vi "FPGAcode_check_values.vi"() -> ()   [LabVIEW 2015]
uses:
  <vilib>/Platform/TimedLoop/XDataNode/wakeup.ctl
  <vilib>/Platform/TimedLoop/XDataNode/XDNodeRunTimeDep.lvlib
  <vilib>/Platform/TimedLoop/XDataNode/nitl_modes.ctl
  <vilib>/Platform/TimedLoop/XDataNode/timing_clust.ctl
  <vilib>/Platform/TimedLoop/XDataNode/XDataNode.xnode
  <vilib>/eio/EIONode/EIONode.xnode
  <vilib>/rvi/eio/common/nirviEmuTemplateMethod_errors.vi
panel:
  out "Check Data?":bool
  out "Filter":i16
  out "Wait time 7":i32
  out "Wait time 6":i32
  out "delay 7":i32
  out "delay 6":i32
  out "Vel Count 7":i32
  out "Vel Count 6":i32
  out "Wait time 5":i32
  out "delay 5":i32
  out "Vel Count 5":i32
  out "Vel Count 4":i32
  out "delay 4":i32
  out "Wait time 4":i32
  out "Vel Count 3":i32
  out "delay 3":i32
  out "Wait time 3":i32
  out "Wait time 2":i32
  out "delay 2":i32
  out "Vel Count 2":i32
  out "Wait time 1":i32
  out "delay 1":i32
  out "Vel Count 1":i32
  out "Filter 1 Detector 3 Correlation":i32
  in  "Filter 2 threshold":i32=1000
  out "Filter 2 Detector 3 Correlation":i32
  in  "Filter 1 threshold":i32=1000
  in  "Filter 3 threshold":i32=1000
  out "Filter 3 Detector 3 Correlation":i32
  in  "Filter 4 threshold":i32=1000
  out "Filter 4 Detector 3 Correlation":i32
  in  "Filter 5 threshold":i32
  out "Filter 5 Detector 3 Correlation":i32
  in  "Filter 6 threshold":i32
  out "Filter 6 Detector 3 Correlation":i32
  in  "Filter 7 threshold":i32
  out "Filter 7 Detector 3 Correlation":i32
  out "Plates":bool
  in  "High Charge Limit":i16
  in  "Low Charge Limit":i16
  in  "High Velocity Count":i32
  in  "Low Velocity Count":i32
  in  "High Mass Limit":i64
  in  "Low Mass Limit":i64
  in  "Mult1":fxp<+,16,7>
  out "Delay1":bool
  in  "One Shot":bool
  out "Not Armed?":bool
  in  "Reset One Shot":bool
  out "Del Not Armed?":bool
  out "IO Module\\AI 0":i16
  out "IO Module\\AI 1":i16
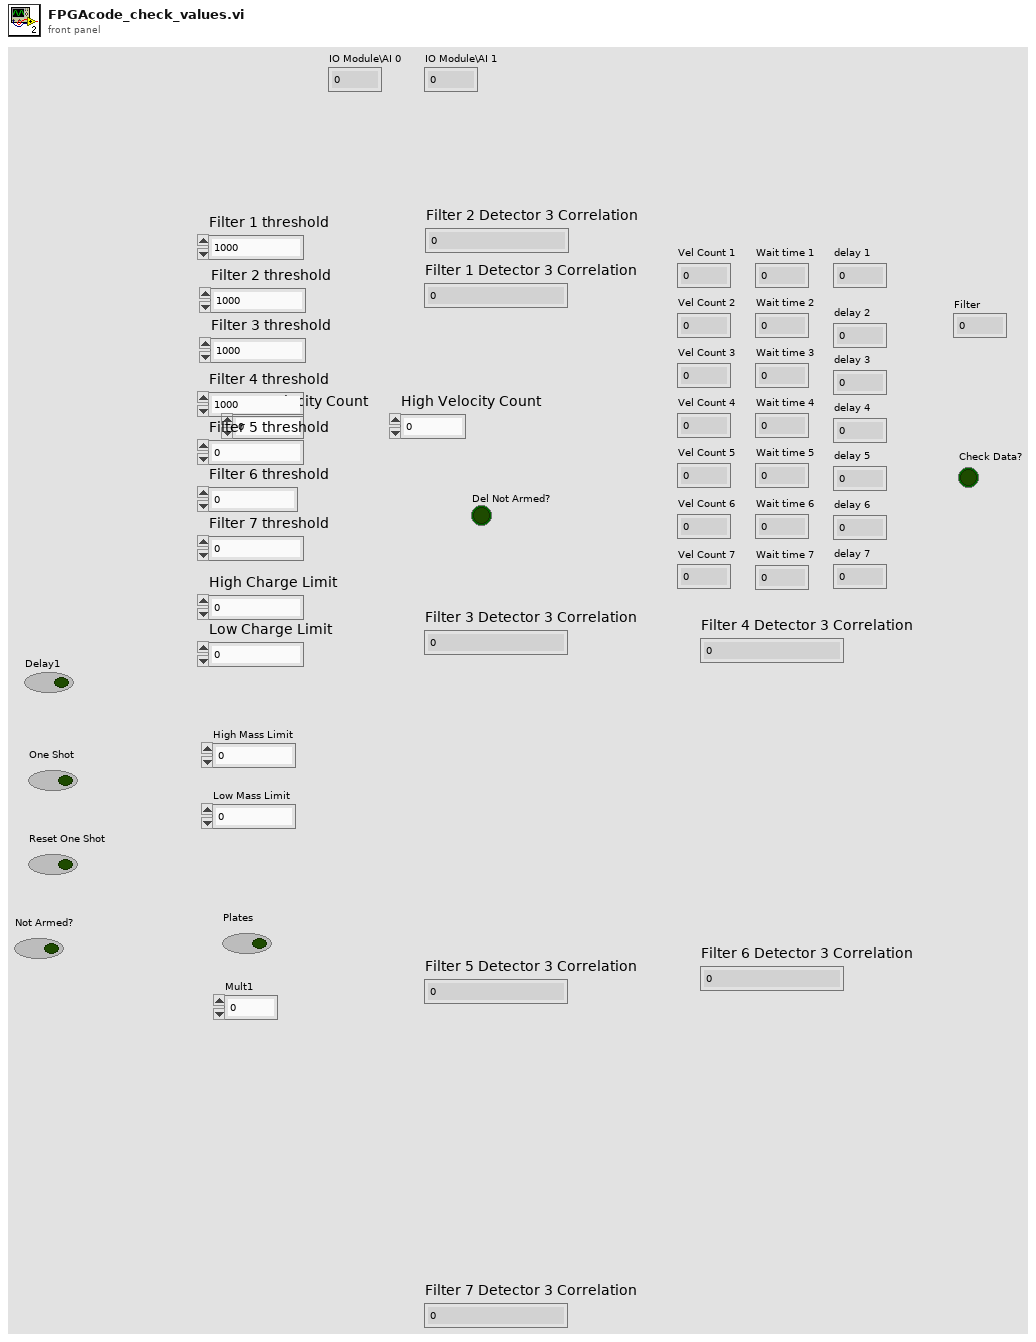
[diagram p1: front panel]
types:
  T1 = typedef "XDNodeRunTimeDep.lvlib/timing_clust.ctl" = cluster{"Expected End [f-1]":u64, "Actual End [f-1]":u64, "Finished Late? [f-1]":bool, "Expected End [i-1]":u64, "Actual End [i-1]":u64, "Finished Late? [i-1]":bool, "Expected Start [i]":u64, "Actual Start [i]":u64, "Expected Start [f]":u64, "Actual Start [f]":u64, "Source Name":string, "Structure Name":string, "Period":i64, "Deadline":i64, "Offset":i64, "Start":i64, "Priority":i32, "Timeout":i32, "Mode":T2, "Wakeup Reason":T3, "Error":errorcluster, "Source Type":string, "Secondary Source Type":string, "Global End Time":u64, "Global Start Time":u64, "Frame Duration":u64, "Iteration Duration":u64, "Assigned CPU":i32, "I/O Scan Engine Mode":u32}
  T2 = typedef "XDNodeRunTimeDep.lvlib/nitl_modes.ctl" = enum32{"No Change", "Process missed periods, maintain original phase", "Discard missed periods, maintain original phase", "Process missed periods, ignore original phase", "Discard missed periods, ignore original phase"}
  T3 = typedef "XDNodeRunTimeDep.lvlib/wakeup.ctl" = enum32{"Normal", "Aborted", "Asynchronous wakeup", "Timing source error", "Timed loop error", "Timeout"}
  T4 = cluster{"Separation cut off 1":i32, "Filter Number":i32, "Separation cut off 2":i32}
  T5 = cluster{"Old Average":i32, "New Average":i32, "Current State":u8, "Detector 1 Correlation":i32, "Detector 3 Correlation":i32, "Velocity Count":i32, "Detector Counter in":i32, "Timeout Count in":i32, "Measured Charge in":i32, "Filter Threshold":i32, "High Correlation in":i32, "Offset":i32, "Offset Average":i32, "Measured Velocity In":i32, "Mult Cluster":cluster{"Mult1":fxp<+,16,7>, "Mult1 Use?":bool}, "Final Delay Count In":u16, "Delay1 In":i32}
  T6 = cluster{"High Charge Limit":i16, "Low Charge Limit":i16, "Low Velocity Count":i32, "High Velocity Count":i32, "Low Velocity Count":i32, fxp<+,30,25>, "High Mass Limit":i64, "Low Mass Limit":i64}
  T7 = cluster{"Average Out":i32, "Next State":u8, "Velocity Count out":i32, "Detector counter out":i32, "Timeout count out":u32, "Measured Charge Out":i32, "High Correlation Out":i32, "Plates":bool, "Offset Out":i32, "Measured Velocity Out":i32, "Final Delay Count Out":u16, "Out1":bool, "Delay1":i32}
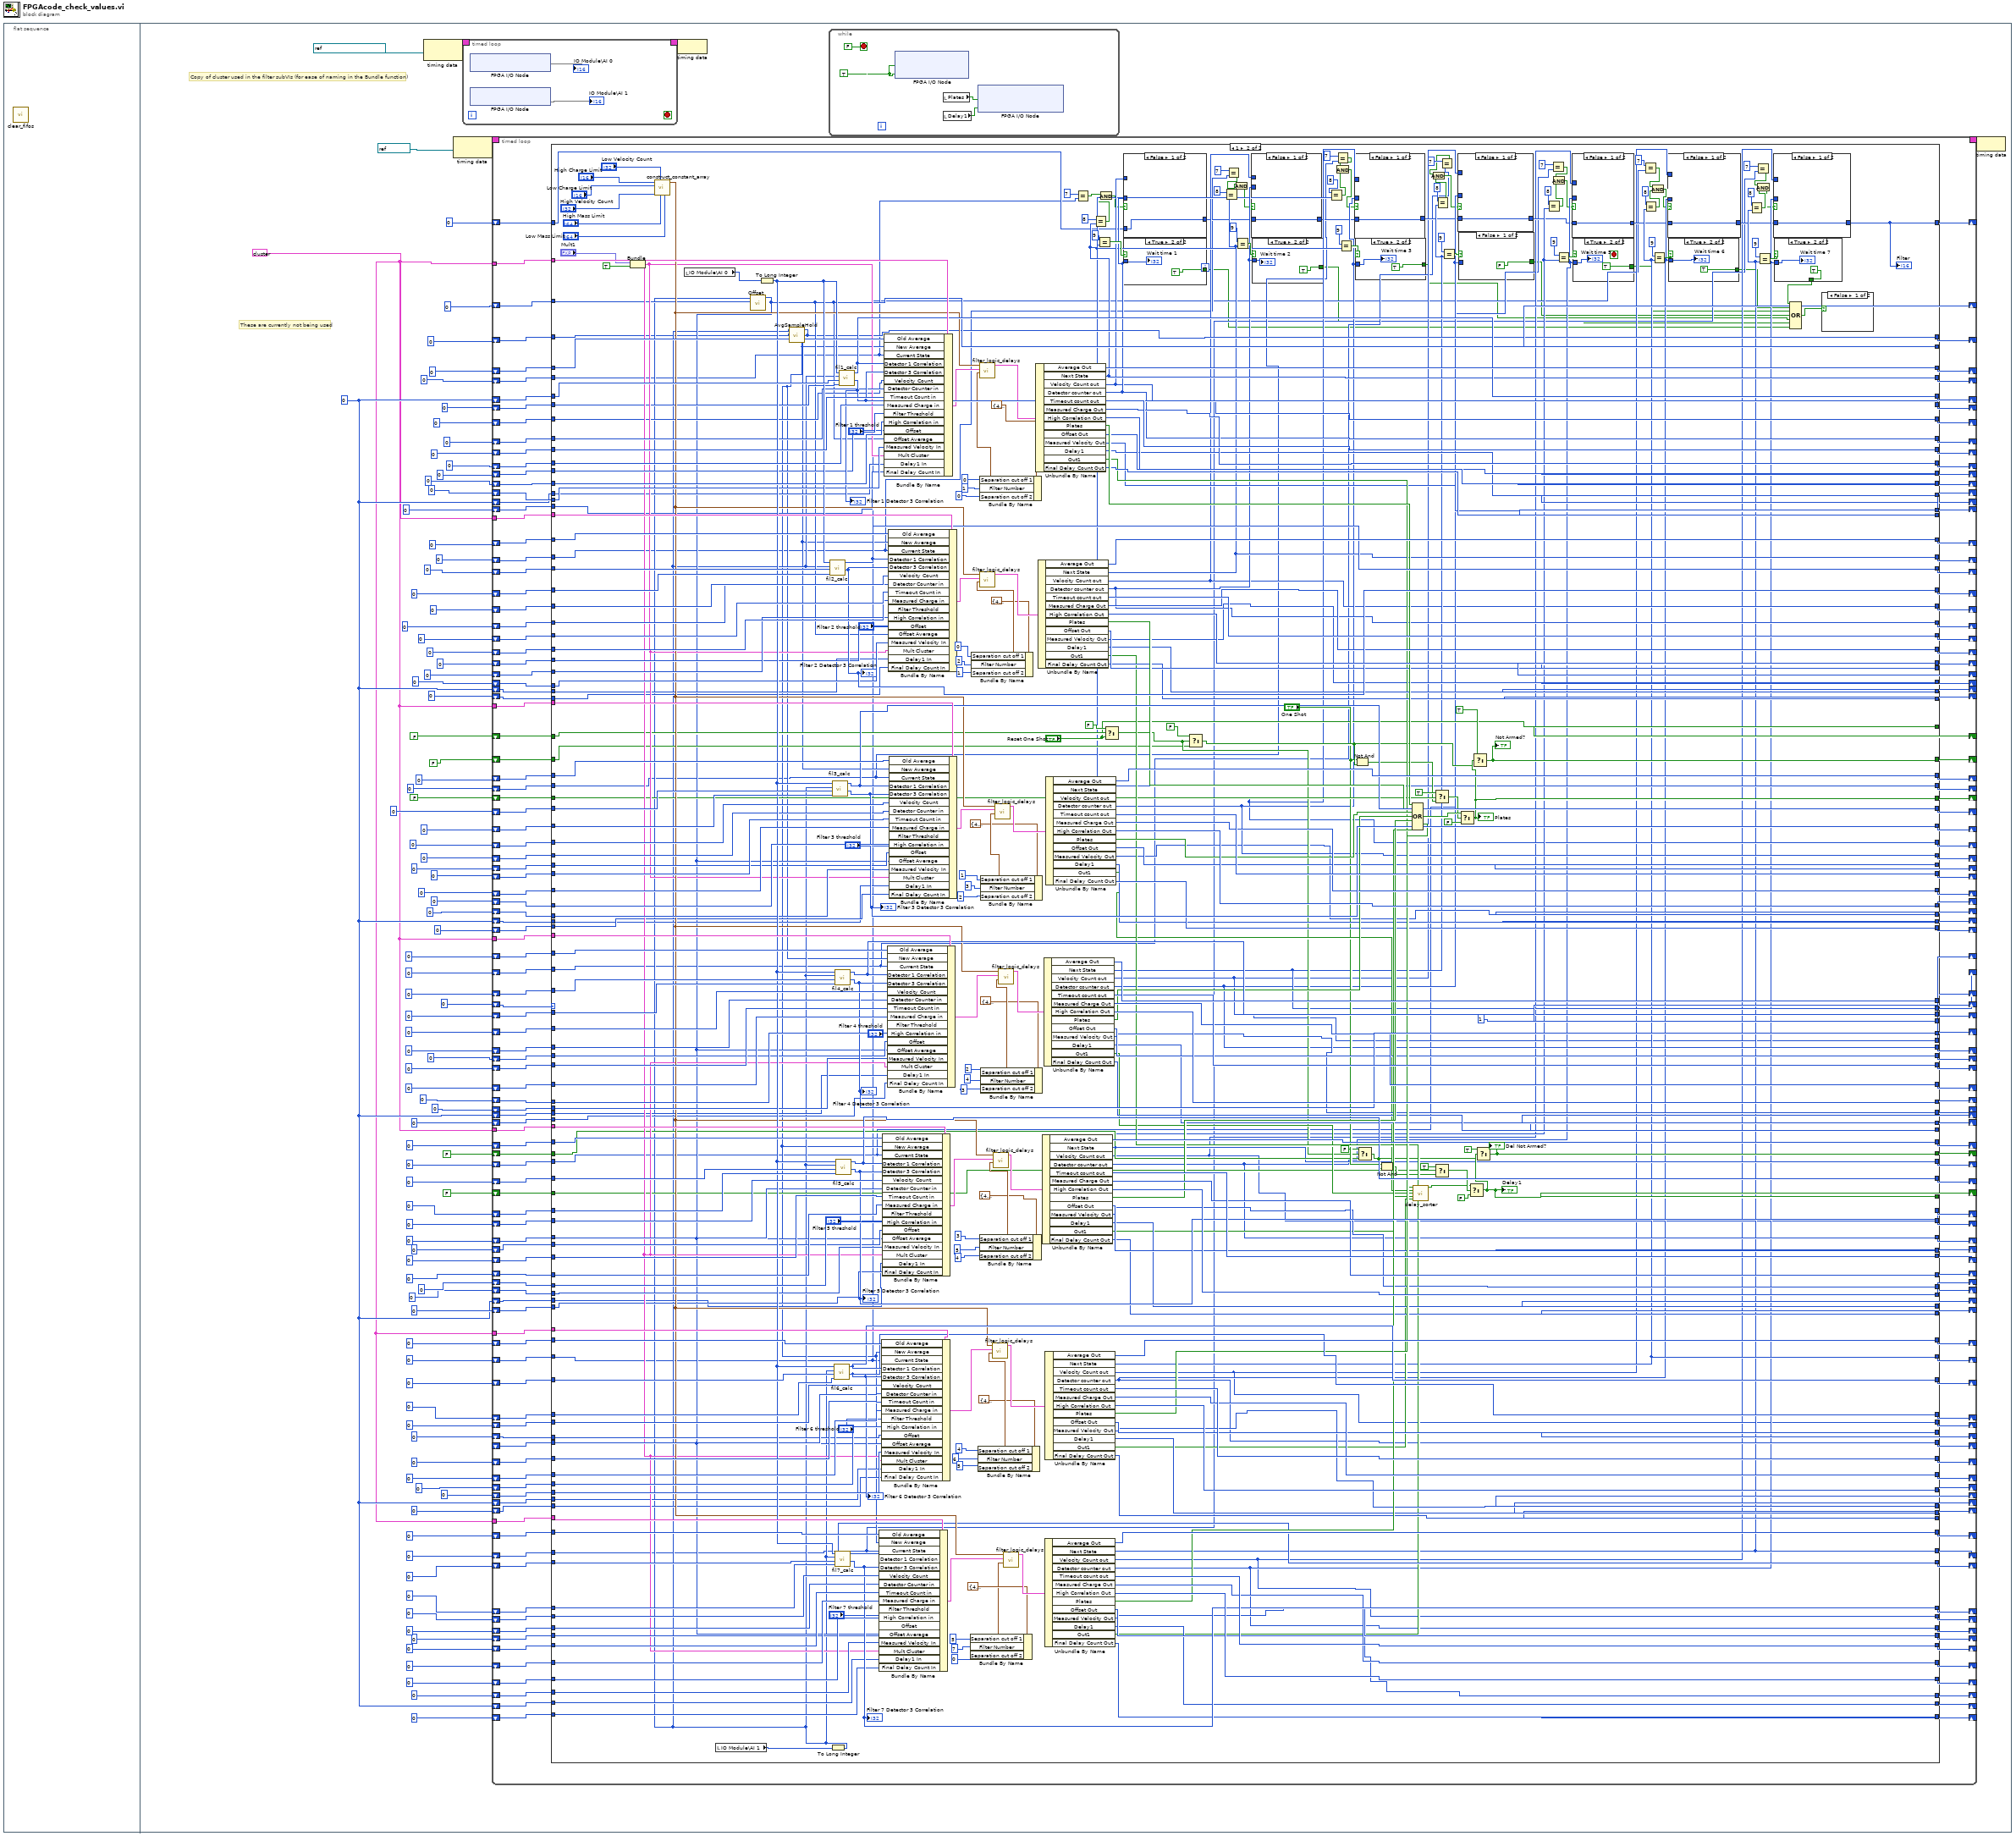
[diagram p0: block diagram]
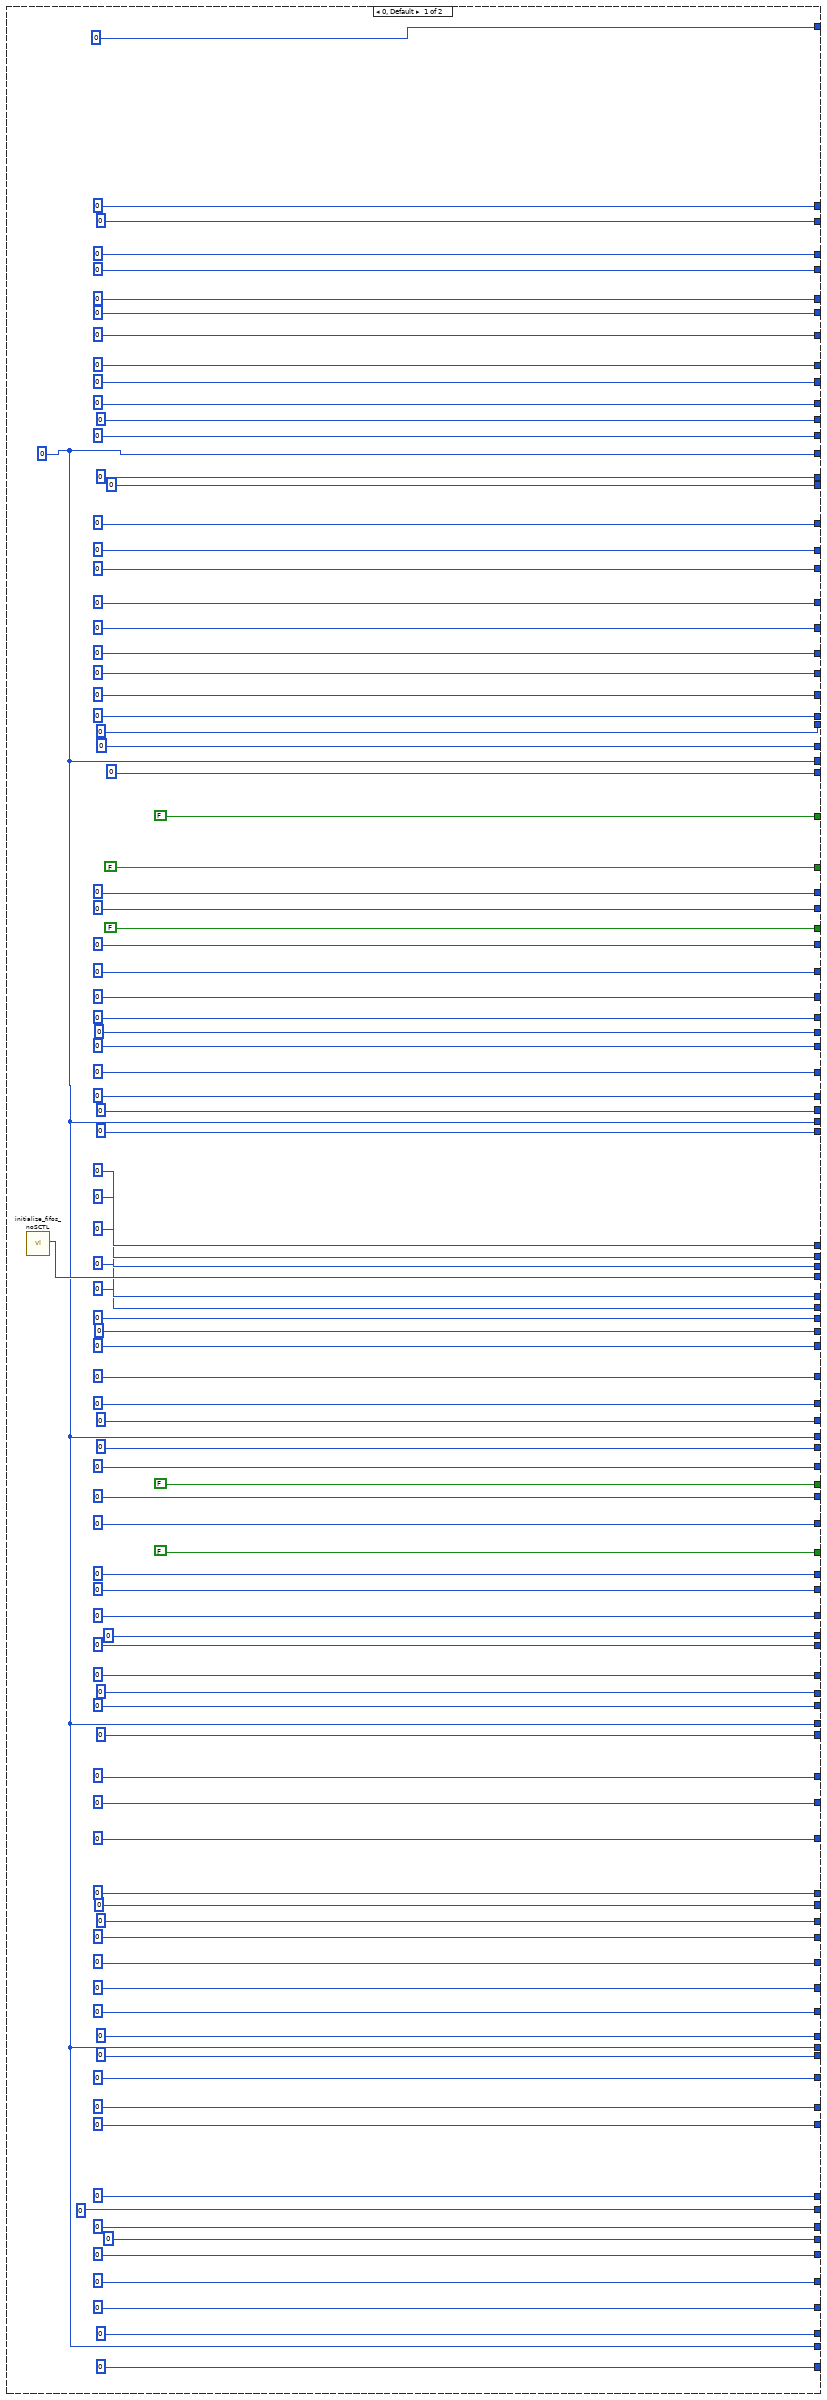
[diagram p2: hidden frame]
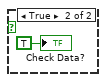
[diagram p3: hidden frame]
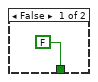
[diagram p4: hidden frame]
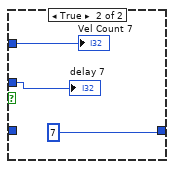
[diagram p5: hidden frame]
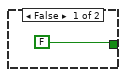
[diagram p6: hidden frame]
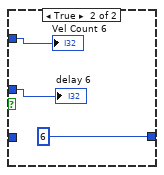
[diagram p7: hidden frame]
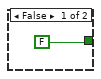
[diagram p8: hidden frame]
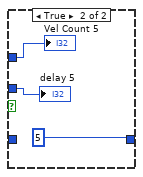
[diagram p9: hidden frame]
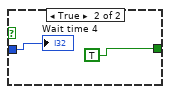
[diagram p10: hidden frame]
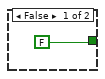
[diagram p11: hidden frame]
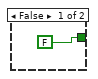
[diagram p12: hidden frame]
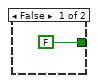
[diagram p13: hidden frame]
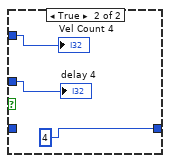
[diagram p14: hidden frame]
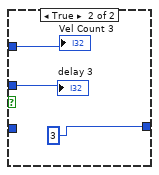
[diagram p15: hidden frame]
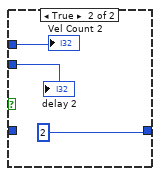
[diagram p16: hidden frame]
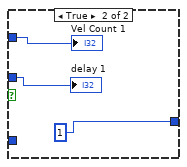
[diagram p17: hidden frame]
diagram:
  n1 = flat-sequence {
    frame #0 {
      n2 = call "clear_fifos.vi"() -> ()  [unwired: 1 in]
    }
    frame #1 {
      w6 = T5 {"Old Average"=0, "New Average"=0, "Current State"=0, "Detector 1 Correlation"=0, "Detector 3 Correlation"=0, "Velocity Count"=0, "Detector Counter in"=0, "Timeout Count in"=0, "Measured Charge in"=0, "Filter Threshold"=0, "High Correlation in"=0, "Offset"=0, "Offset Average"=0, "Measured Velocity In"=0, "Mult Cluster"={"Mult1"=0.0, "Mult1 Use?"=FALSE}, "Final Delay Count In"=0, "Delay1 In"=0} ("Variables Cluster")
      w9 = 0 ("Detector 1 Correlation Out")
      # "These are currently not being used"
      # "Copy of cluster used in the filter subVIs (for ease of naming in the Bundle function)"
      n3 = node-c288(refnum<k21> "IO Module\\Data Clock" ("Source Name")) -> (w35:T1)
      n4 = node-c288(refnum<k21> "26MHz" ("Source Name")) -> (w99:T1)
      n5 = timed-loop {
        timing: w35 -> [_]
        timing-out: [_] -> w34
        stop <- _ stop-if-true
        n6 = xnode "FPGA I/O Node"() -> ("IO Module\\AI 0 Data N"=→"IO Module\\AI 0")  [unwired: 1 in, 1 out]
        n7 = xnode "FPGA I/O Node"() -> ("IO Module\\AI 1 Data N"=→"IO Module\\AI 1")  [unwired: 1 in, 1 out]
      }
      n8 = timed-loop {
        timing: w99 -> [_]
        timing-out: [_] -> w98
        shift-right: [w311] -> _
        shift-left: 0 ("Velocity Count out") -> [w233]
        shift-right: [w312] -> _
        shift-left: 0 ("Detector 1 Correlation out") -> [w234]
        shift-right: [w198] -> _
        shift-left: 0 ("Detector counter out") -> [w235]
        shift-right: [w229] -> _
        shift-left: 0 ("Next State") -> [w236]
        shift-right: [w197] -> _
        shift-left: 0 ("Detector 3 Correlation out") -> [w232]
        shift-right: [w310] -> _
        shift-left: 0 ("Timeout count out") -> [w231]
        shift-right: [w225] -> _
        shift-left: 0 ("Next State") -> [w228]
        shift-right: [w224] -> _
        shift-left: 0 ("Detector counter out") -> [w227]
        shift-right: [w196] -> _
        shift-left: 0 ("Detector 1 Correlation out") -> [w304]
        shift-right: [w301] -> _
        shift-left: 0 ("Velocity Count out") -> [w303]
        shift-right: [w300] -> _
        shift-left: u32 0 ("Detector 3 Correlation out") -> [w302]
        shift-right: [w295] -> _
        shift-left: 0 ("Timeout count out") -> [w296]
        shift-right: [w219] -> _
        shift-left: 0 ("Next State") -> [w222]
        shift-right: [w194] -> _
        shift-left: 0 ("Detector counter out") -> [w292]
        shift-right: [w290] -> _
        shift-left: 0 ("Detector 1 Correlation out") -> [w291]
        shift-right: [w288] -> _
        shift-left: u32 0 ("Velocity Count out") -> [w289]
        shift-right: [w193] -> _
        shift-left: 0 ("Detector 3 Correlation out") -> [w287]
        shift-right: [w286] -> _
        shift-left: 0 ("Timeout count out") -> [w221]
        shift-right: [w313] -> _
        shift-left: u8 0 ("High Correlation Out") -> [w316]
        shift-right: [w305] -> _
        shift-left: u8 0 ("High Correlation Out") -> [w306]
        shift-right: [w220] -> _
        shift-left: 0 ("High Correlation Out") -> [w223]
        shift-right: [w314] -> _
        shift-left: 0 ("Measured Charge Out") -> [w317]
        shift-right: [w307] -> _
        shift-left: 0 ("Measured Charge Out") -> [w308]
        shift-right: [w294] -> _
        shift-left: u8 0 ("Measured Charge Out") -> [w293]
        shift-right: [w184] -> _
        shift-left: 0 ("Output New Average") -> [w318]
        shift-right: [w230] -> _
        shift-left: w9 -> [w237]
        tunnel: w6 -> [w315]
        shift-right: [w195] -> _
        shift-left: 0 ("High Sample Out") -> [w298]
        shift-right: [w299] -> _
        shift-left: 0 ("High Correlation Out") -> [w226]
        tunnel: w6 -> [w309]
        tunnel: w6 -> [w297]
        shift-right: [w285] -> _
        shift-left: 0 ("Average Out") -> [w284]
        shift-right: [w283] -> _
        shift-left: u8 0 ("Next State") -> [w282]
        shift-right: [w215] -> _
        shift-left: 0 ("Detector 1 Correlation out") -> [w217]
        shift-right: [w214] -> _
        shift-left: 0 ("Detector 3 Correlation out") -> [w216]
        shift-right: [w192] -> _
        shift-left: 0 ("Velocity Count out") -> [w281]
        shift-right: [w280] -> _
        shift-left: 0 ("Detector counter out") -> [w279]
        shift-right: [w278] -> _
        shift-left: u32 0 ("Timeout count out") -> [w277]
        shift-right: [w191] -> _
        shift-left: 0 ("Measured Charge Out") -> [w276]
        shift-right: [w275] -> _
        shift-left: 0 ("High Correlation Out") -> [w218]
        tunnel: w6 -> [w274]
        shift-right: [w272] -> _
        shift-left: 0 ("Average Out") -> [w271]
        shift-right: [w270] -> _
        shift-left: u8 0 ("Next State") -> [w269]
        shift-right: [w210] -> _
        shift-left: 0 ("Detector 1 Correlation out") -> [w213]
        shift-right: [w209] -> _
        shift-left: 0 ("Detector 3 Correlation out") -> [w212]
        shift-right: [w190] -> _
        shift-left: 0 ("Velocity Count out") -> [w268]
        shift-right: [w267] -> _
        shift-left: 0 ("Detector counter out") -> [w266]
        shift-right: [w265] -> _
        shift-left: u32 0 ("Timeout count out") -> [w264]
        shift-right: [w189] -> _
        shift-left: 0 ("Measured Charge Out") -> [w263]
        shift-right: [w262] -> _
        shift-left: 0 ("High Correlation Out") -> [w211]
        tunnel: w6 -> [w273]
        shift-right: [w260] -> _
        shift-left: 0 ("Average Out") -> [w258]
        shift-right: [w259] -> _
        shift-left: u8 0 ("Next State") -> [w255]
        shift-right: [w205] -> _
        shift-left: 0 ("Detector 1 Correlation out") -> [w208]
        shift-right: [w204] -> _
        shift-left: 0 ("Detector 3 Correlation out") -> [w207]
        shift-right: [w187] -> _
        shift-left: 0 ("Velocity Count out") -> [w257]
        shift-right: [w254] -> _
        shift-left: _ -> [w256]
        shift-right: [w253] -> _
        shift-left: u32 0 ("Timeout count out") -> [w252]
        shift-right: [w188] -> _
        shift-left: 0 ("Measured Charge Out") -> [w251]
        shift-right: [w250] -> _
        shift-left: 0 ("High Correlation Out") -> [w206]
        tunnel: w6 -> [w261]
        shift-right: [w248] -> _
        shift-left: 0 ("Average Out") -> [w247]
        shift-right: [w246] -> _
        shift-left: u8 0 ("Next State") -> [w238]
        shift-right: [w200] -> _
        shift-left: 0 ("Detector 1 Correlation out") -> [w203]
        shift-right: [w199] -> _
        shift-left: 0 ("Detector 3 Correlation out") -> [w202]
        shift-right: [w186] -> _
        shift-left: 0 ("Velocity Count out") -> [w245]
        shift-right: [w244] -> _
        shift-left: 0 ("Detector counter out") -> [w243]
        shift-right: [w242] -> _
        shift-left: u32 0 ("Timeout count out") -> [w241]
        shift-right: [w185] -> _
        shift-left: 0 ("Measured Charge Out") -> [w240]
        shift-right: [w239] -> _
        shift-left: 0 ("High Correlation Out") -> [w201]
        tunnel: w6 -> [w249]
        shift-right: [w182] -> _
        shift-left: i16 0 -> [w183]
        shift-right: [w180] -> _
        shift-left: 0 -> [w181]
        shift-right: [w179] -> _
        shift-left: 0 -> [w176]
        shift-right: [w177] -> _
        shift-left: 0 -> [w178]
        shift-right: [w174] -> _
        shift-left: 0 ("Offset Out") -> [w175]
        shift-right: [w173] -> _
        shift-left: 0 ("Offset Out") -> [w172]
        shift-right: [w171] -> _
        shift-left: 0 ("Offset Out") -> [w170]
        shift-right: [w169] -> _
        shift-left: 0 ("Offset Out") -> [w168]
        shift-right: [w167] -> _
        shift-left: 0 ("Offset Out") -> [w166]
        shift-right: [w164] -> _
        shift-left: 0 -> [w165]
        shift-right: [w163] -> _
        shift-left: 0 -> [w152]
        shift-right: [w162] -> _
        shift-left: 0 -> [w153]
        shift-right: [w161] -> _
        shift-left: 0 -> [w154]
        shift-right: [w160] -> _
        shift-left: 0 -> [w155]
        shift-right: [w159] -> _
        shift-left: 0 -> [w156]
        shift-right: [w158] -> _
        shift-left: 0 ("Measured Velocity Out") -> [w157]
        shift-right: [w151] -> _
        shift-left: w9 -> [w149]
        shift-right: [w150] -> _
        shift-left: u32 0 ("Final Delay Count Out") -> [w148]
        shift-right: [w147] -> _
        shift-left: w9 -> [w145]
        shift-right: [w146] -> _
        shift-left: u32 0 ("Final Delay Count Out") -> [w144]
        shift-right: [w143] -> _
        shift-left: w9 -> [w141]
        shift-right: [w142] -> _
        shift-left: u32 0 ("Final Delay Count Out") -> [w140]
        shift-right: [w139] -> _
        shift-left: w9 -> [w137]
        shift-right: [w138] -> _
        shift-left: u32 0 ("Final Delay Count Out") -> [w136]
        shift-right: [w135] -> _
        shift-left: w9 -> [w133]
        shift-right: [w134] -> _
        shift-left: u32 0 ("Final Delay Count Out") -> [w132]
        shift-right: [w131] -> _
        shift-left: w9 -> [w129]
        shift-right: [w130] -> _
        shift-left: u32 0 ("Final Delay Count Out") -> [w128]
        shift-right: [w127] -> _
        shift-left: w9 -> [w125]
        shift-right: [w126] -> _
        shift-left: u32 0 ("Final Delay Count Out") -> [w124]
        shift-right: [w122] -> _
        shift-left: FALSE -> [w123]
        shift-right: [w121] -> _
        shift-left: FALSE ("f") -> [w120]
        shift-right: [w119] -> _
        shift-left: FALSE ("Reset One Shot") -> [w118]
        shift-right: [w114] -> _
        shift-left: FALSE -> [w117]
        shift-right: [w115] -> _
        shift-left: FALSE -> [w116]
        shift-right: [w113] -> _
        shift-left: i16 0 ("Filter") -> [w112]
        stop <- _ stop-if-true
        n9 = case shown="1" w183 {
          tunnel: w318 -> [_ w510]
          tunnel: w317 -> [_ w784]
          tunnel: w316 -> [_ w427]
          tunnel: w315 -> [_ w783]
          tunnel: [0 ("Average Out") w782] -> w314
          tunnel: [u16 0 ("Next State") w506] -> w313
          tunnel: [0 ("Detector counter out") w498] -> w312
          tunnel: [u32 0 ("Timeout count out") w781] -> w311
          tunnel: [0 ("High Correlation Out") w780] -> w310
          tunnel: w309 -> [_ w779]
          tunnel: w308 -> [_ w778]
          tunnel: [0 ("Average Out") w777] -> w307
          tunnel: w306 -> [_ w426]
          tunnel: [u16 0 ("Next State") w496] -> w305
          tunnel: w304 -> [_ w776]
          tunnel: w303 -> [_ w638]
          tunnel: w302 -> [_ w775]
          tunnel: [0 ("Detector counter out") w495] -> w301
          tunnel: [u32 0 ("Timeout count out") w774] -> w300
          tunnel: [0 ("High Correlation Out") w773] -> w299
          tunnel: w298 -> [_ w772]
          tunnel: w297 -> [_ w771]
          tunnel: w296 -> [_ w770]
          tunnel: [0 ("Average Out") w769] -> w295
          tunnel: [u16 0 ("Next State") w493] -> w294
          tunnel: w293 -> [_ w425]
          tunnel: w292 -> [_ w768]
          tunnel: w291 -> [_ w637]
          tunnel: [0 ("Detector counter out") w492] -> w290
          tunnel: w289 -> [_ w767]
          tunnel: [u32 0 ("Timeout count out") w766] -> w288
          tunnel: w287 -> [_ w765]
          tunnel: [0 ("High Correlation Out") w764] -> w286
          tunnel: [0 ("Average Out") w763] -> w285
          tunnel: w284 -> [_ w762]
          tunnel: [u16 0 ("Next State") w478] -> w283
          tunnel: w282 -> [_ w424]
          tunnel: w281 -> [_ w761]
          tunnel: [0 ("Detector counter out") w477] -> w280
          tunnel: w279 -> [_ w636]
          tunnel: [u32 0 ("Timeout count out") w760] -> w278
          tunnel: w277 -> [_ w759]
          tunnel: w276 -> [_ w758]
          tunnel: [0 ("High Correlation Out") w757] -> w275
          tunnel: w274 -> [_ w756]
          tunnel: w273 -> [_ w755]
          tunnel: [0 ("Average Out") w754] -> w272
          tunnel: w271 -> [_ w753]
          tunnel: [u16 0 ("Next State") w476] -> w270
          tunnel: w269 -> [_ w423]
          tunnel: w268 -> [_ w752]
          tunnel: [0 ("Detector counter out") w473] -> w267
          tunnel: w266 -> [_ w635]
          tunnel: [u32 0 ("Timeout count out") w751] -> w265
          tunnel: w264 -> [_ w750]
          tunnel: w263 -> [_ w749]
          tunnel: [0 ("High Correlation Out") w748] -> w262
          tunnel: w261 -> [_ w747]
          tunnel: [0 ("Average Out") w746] -> w260
          tunnel: [u16 0 ("Next State") w472] -> w259
          tunnel: w258 -> [_ w745]
          tunnel: w257 -> [_ w744]
          tunnel: w256 -> [_ w634]
          tunnel: w255 -> [_ w422]
          tunnel: [0 ("Detector counter out") w471] -> w254
          tunnel: [u32 0 ("Timeout count out") w743] -> w253
          tunnel: w252 -> [_ w742]
          tunnel: w251 -> [_ w741]
          tunnel: [0 ("High Correlation Out") w740] -> w250
          tunnel: w249 -> [_ w739]
          tunnel: [0 ("Average Out") w738] -> w248
          tunnel: w247 -> [_ w737]
          tunnel: [u16 0 ("Next State") w470] -> w246
          tunnel: w245 -> [_ w736]
          tunnel: [0 ("Detector counter out") w469] -> w244
          tunnel: w243 -> [_ w633]
          tunnel: [u32 0 ("Timeout count out") w735] -> w242
          tunnel: w241 -> [_ w734]
          tunnel: w240 -> [_ w733]
          tunnel: [0 ("High Correlation Out") w732] -> w239
          tunnel: w238 -> [_ w421]
          tunnel: w237 -> [_ w731]
          tunnel: w236 -> [_ w549]
          tunnel: w235 -> [_ w550]
          tunnel: w234 -> [_ w639]
          tunnel: w233 -> [_ w730]
          tunnel: w232 -> [_ w729]
          tunnel: w231 -> [_ w728]
          tunnel: [0 ("Detector 1 Correlation Out") w727] -> w230
          tunnel: [0 ("Detector 3 Correlation Out") w726] -> w229
          tunnel: w228 -> [_ w725]
          tunnel: w227 -> [_ w724]
          tunnel: w226 -> [_ w723]
          tunnel: [0 ("Detector 1 Correlation Out") w722] -> w225
          tunnel: [0 ("Detector 3 Correlation Out") w721] -> w224
          tunnel: w223 -> [_ w720]
          tunnel: w222 -> [_ w719]
          tunnel: w221 -> [_ w718]
          tunnel: [0 ("Detector 1 Correlation Out") w717] -> w220
          tunnel: [0 ("Detector 3 Correlation Out") w716] -> w219
          tunnel: w218 -> [_ w715]
          tunnel: w217 -> [_ w714]
          tunnel: w216 -> [_ w713]
          tunnel: [0 ("Detector 1 Correlation Out") w712] -> w215
          tunnel: [0 ("Detector 3 Correlation Out") w711] -> w214
          tunnel: w213 -> [_ w710]
          tunnel: w212 -> [_ w709]
          tunnel: w211 -> [_ w708]
          tunnel: [0 ("Detector 1 Correlation Out") w707] -> w210
          tunnel: [0 ("Detector 3 Correlation Out") w706] -> w209
          tunnel: w208 -> [_ w705]
          tunnel: w207 -> [_ w704]
          tunnel: w206 -> [_ w703]
          tunnel: [0 ("Detector 1 Correlation Out") w702] -> w205
          tunnel: [0 ("Detector 3 Correlation Out") w701] -> w204
          tunnel: w203 -> [_ w700]
          tunnel: w202 -> [_ w699]
          tunnel: w201 -> [_ w698]
          tunnel: [0 ("Detector 1 Correlation Out") w584] -> w200
          tunnel: [0 ("Detector 3 Correlation Out") w697] -> w199
          tunnel: [0 ("Velocity Count out") w497] -> w198
          tunnel: [0 ("Measured Charge Out") w696] -> w197
          tunnel: [0 ("Velocity Count out") w474] -> w196
          tunnel: [0 ("Measured Charge Out") w695] -> w195
          tunnel: [0 ("Velocity Count out") w475] -> w194
          tunnel: [0 ("Measured Charge Out") w694] -> w193
          tunnel: [0 ("Velocity Count out") w454] -> w192
          tunnel: [0 ("Measured Charge Out") w693] -> w191
          tunnel: [0 ("Velocity Count out") w452] -> w190
          tunnel: [0 ("Measured Charge Out") w692] -> w189
          tunnel: [0 ("Measured Charge Out") w691] -> w188
          tunnel: [0 ("Velocity Count out") w450] -> w187
          tunnel: [0 ("Velocity Count out") w449] -> w186
          tunnel: [0 ("Measured Charge Out") w690] -> w185
          tunnel: [0 ("Output New Average") w509] -> w184
          tunnel: [w412 i16 1 ("Output State")] -> w182
          tunnel: w181 -> [_ w630]
          tunnel: [0 ("Offset Out") w629] -> w180
          tunnel: [0 ("Offset Out") w628] -> w179
          tunnel: w178 -> [_ w513]
          tunnel: [0 ("Output New Average") w512] -> w177
          tunnel: w176 -> [_ w627]
          tunnel: w175 -> [_ w626]
          tunnel: [0 ("Offset Out") w625] -> w174
          tunnel: [0 ("Offset Out") w624] -> w173
          tunnel: w172 -> [_ w623]
          tunnel: [0 ("Offset Out") w622] -> w171
          tunnel: w170 -> [_ w621]
          tunnel: [0 ("Offset Out") w620] -> w169
          tunnel: w168 -> [_ w619]
          tunnel: [0 ("Offset Out") w618] -> w167
          tunnel: w166 -> [_ w617]
          tunnel: w165 -> [_ w612]
          tunnel: [0 ("Measured Velocity Out") w508] -> w164
          tunnel: [0 ("Measured Velocity Out") w494] -> w163
          tunnel: [0 ("Measured Velocity Out") w491] -> w162
          tunnel: [0 ("Measured Velocity Out") w605] -> w161
          tunnel: [0 ("Measured Velocity Out") w604] -> w160
          tunnel: [0 ("Measured Velocity Out") w603] -> w159
          tunnel: [0 ("Measured Velocity Out") w602] -> w158
          tunnel: w157 -> [_ w611]
          tunnel: w156 -> [_ w610]
          tunnel: w155 -> [_ w609]
          tunnel: w154 -> [_ w608]
          tunnel: w153 -> [_ w607]
          tunnel: w152 -> [_ w606]
          tunnel: [w325 w579] -> w151
          tunnel: [u32 0 ("Final Delay Count Out") w597] -> w150
          tunnel: w149 -> [_ w596]
          tunnel: w148 -> [_ w595]
          tunnel: [w325 w594] -> w147
          tunnel: [u32 0 ("Final Delay Count Out") w593] -> w146
          tunnel: w145 -> [_ w592]
          tunnel: w144 -> [_ w591]
          tunnel: [w325 w578] -> w143
          tunnel: [u32 0 ("Final Delay Count Out") w590] -> w142
          tunnel: w141 -> [_ w571]
          tunnel: w140 -> [_ w589]
          tunnel: [w325 w577] -> w139
          tunnel: [u32 0 ("Final Delay Count Out") w588] -> w138
          tunnel: w137 -> [_ w570]
          tunnel: w136 -> [_ w587]
          tunnel: [w325 w576] -> w135
          tunnel: [u32 0 ("Final Delay Count Out") w586] -> w134
          tunnel: w133 -> [_ w569]
          tunnel: w132 -> [_ w585]
          tunnel: [w325 w575] -> w131
          tunnel: [u32 0 ("Final Delay Count Out") w583] -> w130
          tunnel: w129 -> [_ w568]
          tunnel: w128 -> [_ w582]
          tunnel: [w325 w574] -> w127
          tunnel: [u32 0 ("Final Delay Count Out") w581] -> w126
          tunnel: w125 -> [_ w567]
          tunnel: w124 -> [_ w580]
          tunnel: w123 -> [_ w515]
          tunnel: [FALSE ("t") w535] -> w122
          tunnel: [FALSE ("f") w547] -> w121
          tunnel: w120 -> [_ w546]
          tunnel: [FALSE ("Reset One Shot") "Reset One Shot"] -> w119
          tunnel: w118 -> [_ w533]
          tunnel: w117 -> [_ w516]
          tunnel: w116 -> [_ w522]
          tunnel: [FALSE ("Delay1") w521] -> w115
          tunnel: [FALSE w518] -> w114
          tunnel: [i16 0 ("Filter") w461] -> w113
          tunnel: w112 -> [_ w462]
          frame 0, Default {
            w325 = 0
            n10 = call "initialize_fifos_noSCTL.vi"() -> ("Output State"=w412:i16)  [unwired: 11 in]
          }
          frame 1 {
            n11 = Bundle("Mult1"="Mult1", TRUE) -> (w598:cluster{"Mult1":fxp<+,16,7>, bool})  [unwired: 1 in]
            n12 = call "construct_constant_array.vi"("Low Mass Limit"="Low Mass Limit", "High Mass Limit"="High Mass Limit", "Low Velocity Count"="Low Velocity Count", "High Velocity Count"="High Velocity Count", "Low Charge Limit"="Low Charge Limit", "High Charge Limit"="High Charge Limit") -> ("constants cluster"=w599:T6)  [unwired: 5 in]
            n13 = local read "IO Module\\AI 0"() -> (w632:i16)
            n14 = local read "IO Module\\AI 1"() -> (w631:i16)
            n15 = To Long Integer(number=w632) -> (32bit integer=w648:i32)
            n16 = To Long Integer(number=w631) -> (32bit integer=w511:i32)
            n17 = call "Offset.vi"("Previous Average"=w513, "Input Value"=w511) -> ("Output New Average"=w512:i32)  [unwired: 9 in]
            n18 = call "AvgSampleHold.vi"("Previous Average"=w510, "Input Value"=w511) -> ("Output New Average"=w509:i32)  [unwired: 9 in]
            n19 = call "fil2_calc.vi"("Detector 3 Correlation In"=w724, "Detector 1 Correlation In"=w725, "AI1"=w511, "AI0"=w648) -> ("Detector 3 Correlation Out"=w721:i32, "Detector 1 Correlation Out"=w722:i32)  [unwired: 4 in]
            "Filter 2 Detector 3 Correlation" <- w721
            n20 = call "fil3_calc.vi"("Detector 3 Correlation In"=w719, "Detector 1 Correlation In"=w720, "AI1"=w511, "AI0"=w648) -> ("Detector 3 Correlation Out"=w716:i32, "Detector 1 Correlation Out"=w717:i32)  [unwired: 4 in]
            "Filter 3 Detector 3 Correlation" <- w716
            n21 = call "fil6_calc.vi"("Detector 3 Correlation In"=w704, "Detector 1 Correlation In"=w705, "AI1"=w511, "AI0"=w648) -> ("Detector 3 Correlation Out"=w701:i32, "Detector 1 Correlation Out"=w702:i32)  [unwired: 4 in]
            "Filter 6 Detector 3 Correlation" <- w701
            n22 = call "fil4_calc.vi"("Detector 3 Correlation In"=w713, "Detector 1 Correlation In"=w714, "AI1"=w511, "AI0"=w648) -> ("Detector 3 Correlation Out"=w711:i32, "Detector 1 Correlation Out"=w712:i32)  [unwired: 4 in]
            "Filter 4 Detector 3 Correlation" <- w711
            n23 = call "fil7_calc.vi"("Detector 3 Correlation In"=w699, "Detector 1 Correlation In"=w700, "AI1"=w511, "AI0"=w648) -> ("Detector 3 Correlation Out"=w697:i32, "Detector 1 Correlation Out"=w584:i32)  [unwired: 4 in]
            "Filter 7 Detector 3 Correlation" <- w697
            n24 = call "fil5_calc.vi"("Detector 3 Correlation In"=w709, "Detector 1 Correlation In"=w710, "AI1"=w511, "AI0"=w648) -> ("Detector 3 Correlation Out"=w706:i32, "Detector 1 Correlation Out"=w707:i32)  [unwired: 4 in]
            "Filter 5 Detector 3 Correlation" <- w706
            n25 = call "fil1_calc.vi"("Detector 3 Correlation In"=w549, "Detector 1 Correlation In"=w731, "AI1"=w511, "AI0"=w648) -> ("Detector 3 Correlation Out"=w726:i32, "Detector 1 Correlation Out"=w727:i32)  [unwired: 4 in]
            "Filter 1 Detector 3 Correlation" <- w726
            n26 = Bundle By Name(cluster=w739, "Old Average"=w737, "New Average"=w509, "Current State"=w421, "Detector 1 Correlation"=w584, "Detector 3 Correlation"=w697, "Velocity Count"=w736, "Detector Counter in"=w633, "Timeout Count in"=w734, "Measured Charge in"=w733, "Filter Threshold"="Filter 7 threshold", "High Correlation in"=w698, "Offset"=w617, "Offset Average"=w512, "Measured Velocity In"=w611, "Mult Cluster"=w598, "Delay1 In"=w567, "Final Delay Count In"=w580) -> (w537:T5)
            n27 = Bundle By Name(cluster=w747, "Old Average"=w745, "New Average"=w509, "Current State"=w422, "Detector 1 Correlation"=w702, "Detector 3 Correlation"=w701, "Velocity Count"=w744, "Detector Counter in"=w634, "Timeout Count in"=w742, "Measured Charge in"=w741, "Filter Threshold"="Filter 6 threshold", "High Correlation in"=w703, "Offset"=w619, "Offset Average"=w512, "Measured Velocity In"=w610, "Mult Cluster"=w598, "Delay1 In"=w568, "Final Delay Count In"=w582) -> (w538:T5)
            n28 = Bundle By Name(cluster=w755, "Old Average"=w753, "New Average"=w509, "Current State"=w423, "Detector 1 Correlation"=w707, "Detector 3 Correlation"=w706, "Velocity Count"=w752, "Detector Counter in"=w635, "Timeout Count in"=w750, "Measured Charge in"=w749, "Filter Threshold"="Filter 5 threshold", "High Correlation in"=w708, "Offset"=w621, "Offset Average"=w512, "Measured Velocity In"=w609, "Mult Cluster"=w598, "Delay1 In"=w569, "Final Delay Count In"=w585) -> (w539:T5)
            n29 = Bundle By Name(cluster=w783, "Old Average"=w784, "New Average"=w509, "Current State"=w427, "Detector 1 Correlation"=w727, "Detector 3 Correlation"=w726, "Velocity Count"=w550, "Detector Counter in"=w639, "Timeout Count in"=w730, "Measured Charge in"=w729, "Filter Threshold"="Filter 1 threshold", "High Correlation in"=w728, "Offset"=w630, "Offset Average"=w512, "Measured Velocity In"=w612, "Mult Cluster"=w598, "Delay1 In"=w596, "Final Delay Count In"=w595) -> (w543:T5)
            n30 = Bundle By Name(cluster=w756, "Old Average"=w762, "New Average"=w509, "Current State"=w424, "Detector 1 Correlation"=w712, "Detector 3 Correlation"=w711, "Velocity Count"=w761, "Detector Counter in"=w636, "Timeout Count in"=w759, "Measured Charge in"=w758, "Filter Threshold"="Filter 4 threshold", "High Correlation in"=w715, "Offset"=w623, "Offset Average"=w512, "Measured Velocity In"=w608, "Mult Cluster"=w598, "Delay1 In"=w570, "Final Delay Count In"=w587) -> (w540:T5)
            n31 = Bundle By Name(cluster=w779, "Old Average"=w778, "New Average"=w509, "Current State"=w426, "Detector 1 Correlation"=w722, "Detector 3 Correlation"=w721, "Velocity Count"=w776, "Detector Counter in"=w638, "Timeout Count in"=w775, "Measured Charge in"=w772, "Filter Threshold"="Filter 2 threshold", "High Correlation in"=w723, "Offset"=w627, "Offset Average"=w512, "Measured Velocity In"=w606, "Mult Cluster"=w598, "Delay1 In"=w592, "Final Delay Count In"=w591) -> (w542:T5)
            n32 = Bundle By Name(cluster=w771, "Old Average"=w770, "New Average"=w509, "Current State"=w425, "Detector 1 Correlation"=w717, "Detector 3 Correlation"=w716, "Velocity Count"=w768, "Detector Counter in"=w637, "Timeout Count in"=w767, "Measured Charge in"=w765, "Filter Threshold"="Filter 3 threshold", "High Correlation in"=w718, "Offset"=w626, "Offset Average"=w512, "Measured Velocity In"=w607, "Mult Cluster"=w598, "Delay1 In"=w571, "Final Delay Count In"=w589) -> (w541:T5)
            n33 = Bundle By Name(cluster=T4 {"Separation cut off 1"=4, "Filter Number"=5, "Separation cut off 2"=6} ("Filter Specific Constants"), "Separation cut off 1"=5, "Filter Number"=7, "Separation cut off 2"=0) -> (w553:T4)
            n34 = Bundle By Name(cluster=T4 {"Separation cut off 1"=4, "Filter Number"=5, "Separation cut off 2"=6} ("Filter Specific Constants"), "Separation cut off 1"=0, "Filter Number"=2, "Separation cut off 2"=1) -> (w681:T4)
            n35 = Bundle By Name(cluster=T4 {"Separation cut off 1"=4, "Filter Number"=5, "Separation cut off 2"=6} ("Filter Specific Constants"), "Separation cut off 1"=4, "Filter Number"=6, "Separation cut off 2"=5) -> (w671:T4)
            n36 = call "filter_logic_delays.vi"("Filter Specific Constants"=w681, "Variables Cluster"=w542, "controls cluster"=w599) -> ("Output Cluster"=w688:T7)  [unwired: 8 in]
            n37 = Bundle By Name(cluster=T4 {"Separation cut off 1"=4, "Filter Number"=5, "Separation cut off 2"=6} ("Filter Specific Constants"), "Separation cut off 1"=3, "Filter Number"=5, "Separation cut off 2"=4) -> (w673:T4)
            n38 = Bundle By Name(cluster=T4 {"Separation cut off 1"=4, "Filter Number"=5, "Separation cut off 2"=6} ("Filter Specific Constants"), "Separation cut off 1"=0, "Filter Number"=1, "Separation cut off 2"=0) -> (w679:T4)
            n39 = call "filter_logic_delays.vi"("Filter Specific Constants"=w679, "Variables Cluster"=w543, "controls cluster"=w599) -> ("Output Cluster"=w678:T7)  [unwired: 8 in]
            n40 = Bundle By Name(cluster=T4 {"Separation cut off 1"=4, "Filter Number"=5, "Separation cut off 2"=6} ("Filter Specific Constants"), "Separation cut off 1"=1, "Filter Number"=3, "Separation cut off 2"=2) -> (w677:T4)
            n41 = Bundle By Name(cluster=T4 {"Separation cut off 1"=4, "Filter Number"=5, "Separation cut off 2"=6} ("Filter Specific Constants"), "Separation cut off 1"=2, "Filter Number"=4, "Separation cut off 2"=3) -> (w675:T4)
            n42 = call "filter_logic_delays.vi"("Filter Specific Constants"=w671, "Variables Cluster"=w538, "controls cluster"=w599) -> ("Output Cluster"=w670:T7)  [unwired: 8 in]
            n43 = call "filter_logic_delays.vi"("Filter Specific Constants"=w673, "Variables Cluster"=w539, "controls cluster"=w599) -> ("Output Cluster"=w672:T7)  [unwired: 8 in]
            n44 = call "filter_logic_delays.vi"("Filter Specific Constants"=w677, "Variables Cluster"=w541, "controls cluster"=w599) -> ("Output Cluster"=w676:T7)  [unwired: 8 in]
            n45 = call "filter_logic_delays.vi"("Filter Specific Constants"=w675, "Variables Cluster"=w540, "controls cluster"=w599) -> ("Output Cluster"=w674:T7)  [unwired: 8 in]
            n46 = call "filter_logic_delays.vi"("Filter Specific Constants"=w553, "Variables Cluster"=w537, "controls cluster"=w599) -> ("Output Cluster"=w680:T7)  [unwired: 8 in]
            n47 = Unbundle By Name(w678) -> ("Average Out"=w782:i32, "Next State"=w506:u8, "Velocity Count out"=w497:i32, "Detector counter out"=w498:i32, "Timeout count out"=w781:u32, "Measured Charge Out"=w696:i32, "High Correlation Out"=w780:i32, "Plates"=w646:bool, "Offset Out"=w629:i32, "Measured Velocity Out"=w508:i32, "Delay1"=w579:i32, "Out1"=w573:bool, "Final Delay Count Out"=w597:u16)
            n48 = Unbundle By Name(w688) -> ("Average Out"=w777:i32, "Next State"=w496:u8, "Velocity Count out"=w474:i32, "Detector counter out"=w495:i32, "Timeout count out"=w774:u32, "Measured Charge Out"=w695:i32, "High Correlation Out"=w773:i32, "Plates"=w645:bool, "Offset Out"=w628:i32, "Measured Velocity Out"=w494:i32, "Delay1"=w594:i32, "Out1"=w572:bool, "Final Delay Count Out"=w593:u16)
            n49 = Unbundle By Name(w672) -> ("Average Out"=w754:i32, "Next State"=w476:u8, "Velocity Count out"=w452:i32, "Detector counter out"=w473:i32, "Timeout count out"=w751:u32, "Measured Charge Out"=w692:i32, "High Correlation Out"=w748:i32, "Plates"=w642:bool, "Offset Out"=w622:i32, "Measured Velocity Out"=w604:i32, "Delay1"=w576:i32, "Out1"=w563:bool, "Final Delay Count Out"=w586:u16)
            n50 = Unbundle By Name(w674) -> ("Average Out"=w763:i32, "Next State"=w478:u8, "Velocity Count out"=w454:i32, "Detector counter out"=w477:i32, "Timeout count out"=w760:u32, "Measured Charge Out"=w693:i32, "High Correlation Out"=w757:i32, "Plates"=w643:bool, "Offset Out"=w624:i32, "Measured Velocity Out"=w605:i32, "Delay1"=w577:i32, "Out1"=w564:bool, "Final Delay Count Out"=w588:u16)
            n51 = Unbundle By Name(w680) -> ("Average Out"=w738:i32, "Next State"=w470:u8, "Velocity Count out"=w449:i32, "Detector counter out"=w469:i32, "Timeout count out"=w735:u32, "Measured Charge Out"=w690:i32, "High Correlation Out"=w732:i32, "Plates"=w640:bool, "Offset Out"=w618:i32, "Measured Velocity Out"=w602:i32, "Delay1"=w574:i32, "Out1"=w562:bool, "Final Delay Count Out"=w581:u16)
            n52 = Unbundle By Name(w670) -> ("Average Out"=w746:i32, "Next State"=w472:u8, "Velocity Count out"=w450:i32, "Detector counter out"=w471:i32, "Timeout count out"=w743:u32, "Measured Charge Out"=w691:i32, "High Correlation Out"=w740:i32, "Plates"=w641:bool, "Offset Out"=w620:i32, "Measured Velocity Out"=w603:i32, "Delay1"=w575:i32, "Out1"=w561:bool, "Final Delay Count Out"=w583:u16)
            n53 = Unbundle By Name(w676) -> ("Average Out"=w769:i32, "Next State"=w493:u8, "Velocity Count out"=w475:i32, "Detector counter out"=w492:i32, "Timeout count out"=w766:u32, "Measured Charge Out"=w694:i32, "High Correlation Out"=w764:i32, "Plates"=w644:bool, "Offset Out"=w625:i32, "Measured Velocity Out"=w491:i32, "Delay1"=w578:i32, "Out1"=w565:bool, "Final Delay Count Out"=w590:u16)
            n54 = Equal?(x=u16 7, y=w427) -> (x = y?=w428:bool)
            n55 = Equal?(x=u8 8, y=w506) -> (x = y?=w460:bool)
            n56 = Equal?(x=u8 9, y=w506) -> (x = y?=w504:bool)
            n57 = And(x=w428, y=w460) -> (x .and. y?=w459:bool)
            n58 = Select(t=FALSE, s=w533, f="Reset One Shot") -> (s? t:f=w524:bool)
            n59 = case shown="False" w459 {
              tunnel: w498 -> [_ w834]
              tunnel: w497 -> [_ w833]
              tunnel: [w831 i16 1 ("Filter")] -> w468
              tunnel: w462 -> [w831 _]
              frame False {
              }
              frame True {
                "Vel Count 1" <- w833
                "delay 1" <- w834
              }
            }
            n60 = case shown="True" w504 {
              tunnel: w498 -> [_ w818]
              tunnel: [FALSE TRUE] -> w414
              frame False {
              }
              frame True {
                "Wait time 1" <- w818
              }
            }
            n61 = Select(t=FALSE, s=w524, f=w515) -> (s? t:f=w536:bool)
            n62 = Equal?(x=u8 8, y=w496) -> (x = y?=w431:bool)
            n63 = Equal?(x=u16 7, y=w426) -> (x = y?=w430:bool)
            n64 = And(x=w431, y=w430) -> (x .and. y?=w429:bool)
            n65 = Equal?(x=u8 9, y=w496) -> (x = y?=w501:bool)
            n66 = case shown="False" w429 {
              tunnel: w495 -> [_ w830]
              tunnel: w474 -> [_ w829]
              tunnel: w468 -> [w827 _]
              tunnel: [w827 i16 2 ("Filter")] -> w467
              frame False {
              }
              frame True {
                "Vel Count 2" <- w829
                "delay 2" <- w830
              }
            }
            n67 = case shown="True" w501 {
              tunnel: w495 -> [_ w815]
              tunnel: [FALSE TRUE] -> w415
              frame False {
              }
              frame True {
                "Wait time 2" <- w815
              }
            }
            n68 = Equal?(x=u8 8, y=w493) -> (x = y?=w433:bool)
            n69 = Equal?(x=u16 7, y=w425) -> (x = y?=w434:bool)
            n70 = And(x=w434, y=w433) -> (x .and. y?=w432:bool)
            n71 = Equal?(x=u8 9, y=w493) -> (x = y?=w500:bool)
            n72 = case shown="False" w432 {
              tunnel: w492 -> [_ w825]
              tunnel: w475 -> [_ w826]
              tunnel: w467 -> [w823 _]
              tunnel: [w823 i16 3 ("Filter")] -> w466
              frame False {
              }
              frame True {
                "delay 3" <- w825
                "Vel Count 3" <- w826
              }
            }
            n73 = Not And(1:w536, 2:"One Shot") -> (0:w527:bool)
            n74 = case shown="True" w500 {
              tunnel: w492 -> [_ w812]
              tunnel: [FALSE TRUE] -> w416
              frame False {
              }
              frame True {
                "Wait time 3" <- w812
              }
            }
            n75 = Select(t=FALSE, s=w524, f=w516) -> (s? t:f=w519:bool)
            n76 = Not And(1:w519, 2:"One Shot") -> (0:w525:bool)
            n77 = Compound Arithmetic op=OR(w646, w645, w644, w643, w642, w641, w640) -> (w552:bool)
            n78 = call "delay_sorter.vi"("Out1 1"=w573, "Out1 2"=w572, "Out1 3"=w565, "Out1 4"=w564, "Out1 5"=w563, "Out1 6"=w561, "Out1 7"=w562) -> ("Delay1"=w529:bool)  [unwired: 8 in]
            n79 = Select(t=TRUE, s=w546, f=w527) -> (s? t:f=w544:bool)
            n80 = Select(t=TRUE, s=w522, f=w525) -> (s? t:f=w531:bool)
            n81 = Equal?(x=u8 8, y=w478) -> (x = y?=w435:bool)
            n82 = Equal?(x=u16 7, y=w424) -> (x = y?=w437:bool)
            n83 = And(x=w437, y=w435) -> (x .and. y?=w436:bool)
            n84 = Equal?(x=u8 9, y=w478) -> (x = y?=w488:bool)
            n85 = case shown="False" w436 {
              tunnel: w454 -> [_ w822]
              tunnel: w477 -> [_ w821]
              tunnel: w466 -> [w819 _]
              tunnel: [w819 i16 4 ("Filter")] -> w465
              frame False {
              }
              frame True {
                "delay 4" <- w821
                "Vel Count 4" <- w822
              }
            }
            n86 = case shown="False" w488 {
              tunnel: w477 -> [_ w809]
              tunnel: [FALSE TRUE] -> w417
              frame False {
              }
              frame True {
                "Wait time 4" <- w809
              }
            }
            n87 = Select(t=w552, s=w544, f=FALSE) -> (s? t:f=w547:bool)
            "Plates" <- w547
            n88 = Select(t=w529, s=w531, f=FALSE) -> (s? t:f=w521:bool)
            "Delay1" <- w521
            n89 = Select(t=TRUE, s=w547, f=w536) -> (s? t:f=w535:bool)
            "Not Armed?" <- w535
            n90 = Select(t=TRUE, s=w521, f=w519) -> (s? t:f=w518:bool)
            "Del Not Armed?" <- w518
            n91 = Equal?(x=u8 8, y=w476) -> (x = y?=w439:bool)
            n92 = Equal?(x=u16 7, y=w423) -> (x = y?=w440:bool)
            n93 = And(x=w440, y=w439) -> (x .and. y?=w438:bool)
            n94 = Equal?(x=u8 9, y=w476) -> (x = y?=w487:bool)
            n95 = case shown="False" w438 {
              tunnel: w452 -> [_ w806]
              tunnel: w473 -> [_ w805]
              tunnel: w465 -> [w803 _]
              tunnel: [w803 i16 5 ("Filter")] -> w464
              frame False {
              }
              frame True {
                "Vel Count 5" <- w806
                "delay 5" <- w805
              }
            }
            n96 = case shown="True" w487 {
              tunnel: w473 -> [_ w802]
              tunnel: [FALSE TRUE] -> w418
              frame False {
              }
              frame True {
                "Wait time 5" <- w802
              }
            }
            n97 = Equal?(x=u16 7, y=w422) -> (x = y?=w442:bool)
            n98 = Equal?(x=u8 8, y=w472) -> (x = y?=w443:bool)
            n99 = And(x=w442, y=w443) -> (x .and. y?=w441:bool)
            n100 = Equal?(x=u8 9, y=w472) -> (x = y?=w482:bool)
            n101 = case shown="False" w441 {
              tunnel: w450 -> [_ w799]
              tunnel: w471 -> [_ w798]
              tunnel: w464 -> [w796 _]
              tunnel: [w796 i16 6 ("Filter")] -> w463
              frame False {
              }
              frame True {
                "Vel Count 6" <- w799
                "delay 6" <- w798
              }
            }
            n102 = case shown="True" w482 {
              tunnel: w471 -> [_ w795]
              tunnel: [FALSE TRUE] -> w419
              frame False {
              }
              frame True {
                "Wait time 6" <- w795
              }
            }
            n103 = Equal?(x=u8 8, y=w470) -> (x = y?=w446:bool)
            n104 = Equal?(x=u16 7, y=w421) -> (x = y?=w444:bool)
            n105 = And(x=w444, y=w446) -> (x .and. y?=w445:bool)
            n106 = Equal?(x=u8 9, y=w470) -> (x = y?=w481:bool)
            n107 = case shown="False" w445 {
              tunnel: w449 -> [_ w792]
              tunnel: w469 -> [_ w791]
              tunnel: w463 -> [w789 _]
              tunnel: [w789 i16 7 ("Filter")] -> w461
              frame False {
              }
              frame True {
                "Vel Count 7" <- w792
                "delay 7" <- w791
              }
            }
            "Filter" <- w461
            n108 = case shown="True" w481 {
              tunnel: w469 -> [_ w788]
              tunnel: [FALSE TRUE] -> w420
              frame False {
              }
              frame True {
                "Wait time 7" <- w788
              }
            }
            n109 = Compound Arithmetic op=OR(w420, w419, w418, w417, w416, w415, w414) -> (w413:bool)
            n110 = case shown="False" w413 {
              frame False {
              }
              frame True {
                "Check Data?" <- TRUE ("Check Data?")
              }
            }
          }
        }
      }
      n111 = node-c288(w34) -> ()
      n112 = while {
        stop <- FALSE stop-if-true
        w110 = TRUE ("IO Module\\PFI Enable")
        n113 = xnode "FPGA I/O Node"("IO Module\\PFI 0 WE"=w110, "IO Module\\PFI 1 WE"=w110) -> ()  [unwired: 2 in, 2 out]
        n114 = local read "Plates"() -> (w109:bool)
        n115 = local read "Delay1"() -> (w108:bool)
        n116 = xnode "FPGA I/O Node"("IO Module\\PFI 0 Wr Data"=w109, "IO Module\\PFI 1 Wr Data"=w108) -> ()  [unwired: 2 in, 2 out]
      }
      n117 = node-c288(w98) -> ()
    }
  }
